vi "Destroy JKISM Message Event.vi"(8 "error in (no error)":errorcluster, 11 "Module":string) -> (0 "error out":errorcluster)   [LabVIEW 2017, in "JKISM Message Event.lvlib"]
uses:
  JKISM Message Event.lvlib
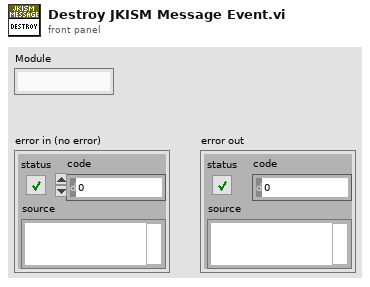
[diagram p1: front panel]
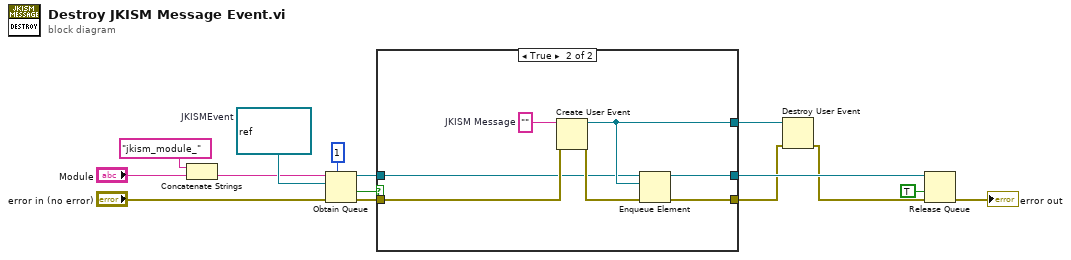
[diagram p0: block diagram]
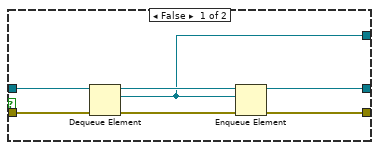
[diagram p2: hidden frame]
diagram:
  w10 = refnum<user-event> refnum  # JKISMEvent
  n1 = Concatenate Strings("jkism_module_" ("string"), "Module") -> (w8:string)
  n2 = Obtain Queue(max queue size (-1, unlimited)=1, name (unnamed)=w8, element data type=w10, error in (no error)="error in (no error)") -> (queue out=w12:refnum<queue>, created new?=w9:bool, error out=w13:errorcluster)  [unwired: 1 in]
  n3 = case shown="True" w9 {
    tunnel: [w19 w29] -> w2
    tunnel: w13 -> [w22 w27]
    tunnel: [w17 w26] -> w3
    tunnel: w12 -> [w20 w25]
    tunnel: [w16 w23] -> w5
    frame False {
      n4 = Dequeue Element(queue=w20, error in (no error)=w22) -> (queue out=w18:refnum<queue>, element=w17:refnum<user-event>, error out=w21:errorcluster)  [unwired: 1 in, 1 out]
      n5 = Enqueue Element(queue=w18, element=w17, error in (no error)=w21) -> (queue out=w16:refnum<queue>, error out=w19:errorcluster)  [unwired: 1 in, 1 out]
    }
    frame True {
      w24 = ""  # JKISM Message
      n6 = Create User Event(user event datatype=w24, error in=w27) -> (user event=w26:refnum<user-event>, error out=w28:errorcluster)
      n7 = Enqueue Element(queue=w25, element=w26, error in (no error)=w28) -> (queue out=w23:refnum<queue>, error out=w29:errorcluster)  [unwired: 1 in, 1 out]
    }
  }
  n8 = Destroy User Event(user event=w3, error in=w2) -> (error out=w1:errorcluster)
  n9 = Release Queue(queue=w5, force destroy? (F)=TRUE, error in (no error)=w1) -> (error out=→"error out":errorcluster)  [unwired: 2 out]
